vi "PositionControlTest.vi"() -> ()   [LabVIEW 2009, in "Test.lvlib"]
uses:
  Test.lvlib
  Drive/Drive_PositionControlMode.ctl
  FPGA.lvlib
  Motor.lvlib
  Drive.lvlib
panel:
  out "error out":errorcluster
  in  "Type":u8
  in  "Speed limit":dbl=0.5
  in  "Y rel (Right)":dbl
  in  "X rel (Left)":dbl
  in  "stop":bool
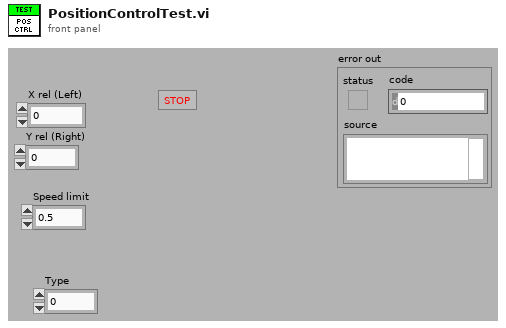
[diagram p1: front panel]
types:
  T1 = typedef "Drive.lvlib/Drive_PositionControlMode.ctl" = enum16{"TurnThenStraight"}
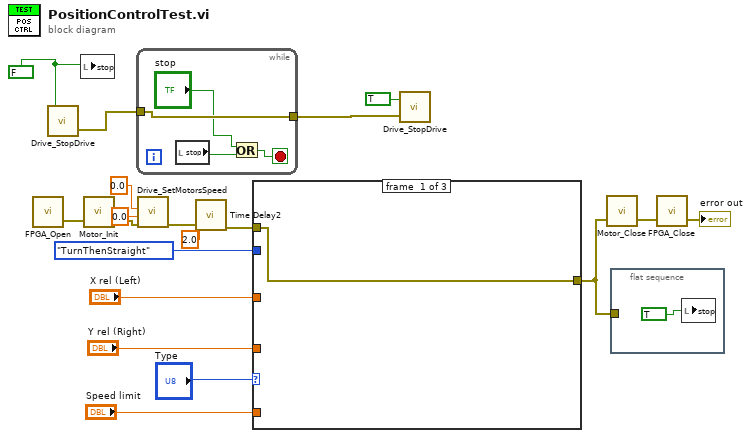
[diagram p0: block diagram]
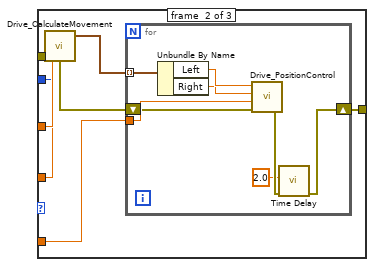
[diagram p2: hidden frame]
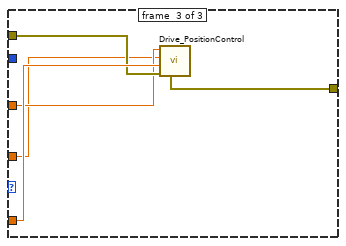
[diagram p3: hidden frame]
diagram:
  w11 = FALSE ("Abort?")
  n1 = call "FPGA_Open.vi"() -> ("error out"=w10:errorcluster)  [unwired: 3 in]
  n2 = call "Drive_StopDrive.vi"("Abort?"=w11) -> ("error out"=w18:errorcluster)  [unwired: 2 in]
  n3 = local write "stop"(w11) -> ()
  n4 = call "Motor_Init.vi"("error in"=w10) -> ("error out"=w6:errorcluster)  [unwired: 2 in]
  n5 = while {
    tunnel: w18 -> [w23]
    tunnel: [w23] -> w17
    stop <- w22 stop-if-true
    n6 = local read "stop"() -> (w21:bool)
    n7 = Or(x="stop", y=w21) -> (x .or. y?=w22:bool)
  }
  n8 = call "Drive_SetMotorsSpeed.vi"("error in"=w6, "Right_Speed"=0.0, "Left_Speed"=0.0) -> ("error out"=w5:errorcluster)  [unwired: 7 in, 1 out]
  n9 = call "Time Delay2"("error in (no error)"=w5, "Delay Time (s)"=2.0) -> ("error out"=w8:errorcluster)  [unwired: 9 in]
  n10 = case shown="2" "Type" {
    tunnel: "X rel (Left)" -> [_ w32 w42]
    tunnel: "Y rel (Right)" -> [_ w31 w41]
    tunnel: Drive_PositionControlMode."TurnThenStraight" ("Mode") -> [_ w30 _]
    tunnel: "Speed limit" -> [_ w27 w45]
    tunnel: [w24 w26 w43] -> w12
    tunnel: w8 -> [w24 w25 w44]
    frame #0 {
    }
    frame #1 {
      n11 = call "Drive_CalculateMovement.vi"("error in"=w25, "Mode"=w30, "Y rel"=w31, "X rel"=w32) -> ("error out"=w28:errorcluster, "Movements"=w29:cluster{"Left":dbl, "Right":dbl}[])  [unwired: 1 in]
      n12 = for {
        tunnel: w29 -> [w39] mode=indexing
        tunnel: w27 -> [w40]
        shift-right: [w34] -> w26
        shift-left: w28 -> [w36]
        n13 = Unbundle By Name(w39) -> ("Left"=w38:dbl, "Right"=w37:dbl)
        n14 = call "Drive_PositionControl.vi"("error in"=w36, "Speed limit"=w40, "Right_Distance"=w37, "Left_Distance"=w38) -> ("error out"=w35:errorcluster)  [unwired: 7 in]
        n15 = call "Time Delay"("error in (no error)"=w35, "Delay Time (s)"=2.0) -> ("error out"=w34:errorcluster)  [unwired: 9 in]
      }
    }
    frame #2 {
      n16 = call "Drive_PositionControl.vi"("error in"=w44, "Speed limit"=w45, "Right_Distance"=w41, "Left_Distance"=w42) -> ("error out"=w43:errorcluster)  [unwired: 7 in]
    }
  }
  n17 = call "Drive_StopDrive.vi"("error in"=w17, "Abort?"=TRUE) -> ()  [unwired: 1 in, 1 out]
  n18 = call "Motor_Close.vi"("error in"=w12) -> ("error out"=w19:errorcluster)  [unwired: 2 in]
  n19 = flat-sequence {
    tunnel: w12 -> [_]
    frame #0 {
      n20 = local write "stop"(TRUE) -> ()
    }
  }
  n21 = call "FPGA_Close.vi"("error in (no error)"=w19) -> ("error out"=→"error out":errorcluster)  [unwired: 2 in]
